vi "Create Electrode Array_2.vi"(7 "Current Channel":string, 8 "Insert\nBreak":bool=TRUE, 9 "Inverse\nPolarity":bool=TRUE, 10 "Electrode number, N":u16=100, 11 "Array Mode":u16(ring) items=["None", "Gradient + Dipole dipole", "Gradient", "Dipole Dipole", "Schlumberger"]) -> (3 "Current Mode":u8[][](array[numeric]))   [LabVIEW 2023]
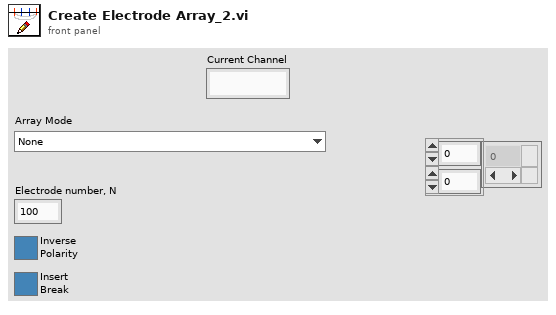
[diagram p1: front panel]
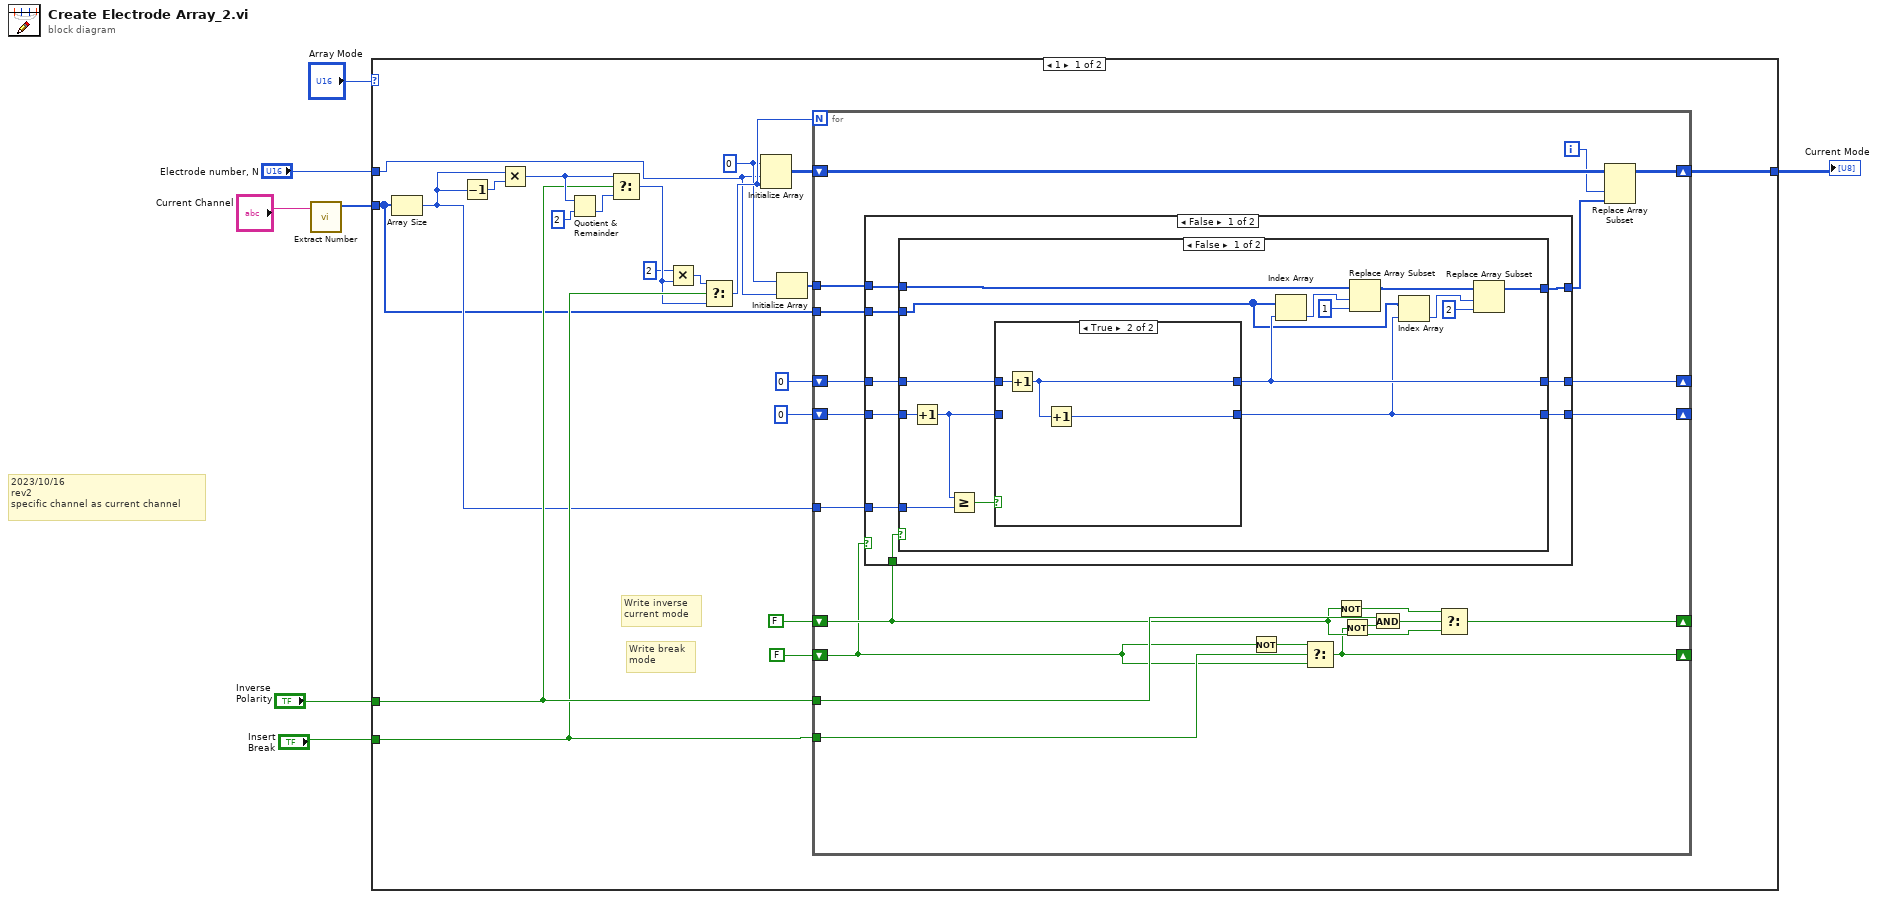
[diagram p0: block diagram]
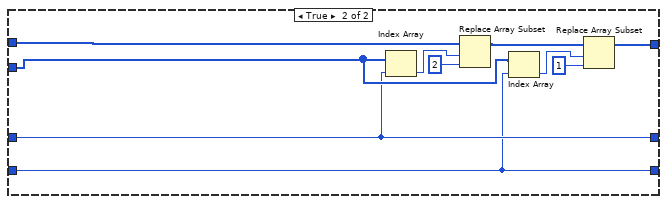
[diagram p3: hidden frame]
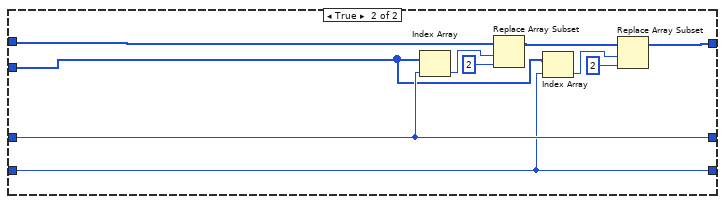
[diagram p4: hidden frame]
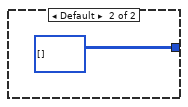
[diagram p5: hidden frame]
diagram:
  # "2023/10/16\nrev2 \nspecific channel as current channel"
  n1 = call "Extract Number.vi"("input string"="Current Channel") -> ("Array"=w1:i32[])  [unwired: 10 in]
  n2 = case shown="1" "Array Mode" {
    tunnel: "Electrode number, N" -> [w10 _]
    tunnel: "Inverse\nPolarity" -> [w18 _]
    tunnel: "Insert\nBreak" -> [w17 _]
    tunnel: [w14 u8[][] []] -> w3
    tunnel: w1 -> [w8 _]
    frame 1 {
      w15 = u8 0 ("stateArray")
      # "Write break\nmode"
      # "Write inverse\ncurrent mode"
      n3 = Array Size(array=w8) -> (size(s)=w9:i32)
      n4 = Decrement(x=w9) -> (x-1=w28:i32)
      n5 = Multiply(x=w9, y=w28) -> (x*y=w27:i32)
      n6 = Quotient & Remainder(x=w27, y=u16 2) -> (floor(x/y)=w25:i32)  [unwired: 1 out]
      n7 = Select(t=w27, s=w18, f=w25) -> (s? t:f=w12:i32)
      n8 = Multiply(x=u16 2, y=w12) -> (x*y=w13:i32)
      n9 = Select(t=w13, s=w17, f=w12) -> (s? t:f=w23:i32)
      n10 = Initialize Array(w15, w10, w23) -> (w24:u8[][])
      n11 = Initialize Array(w15, w10) -> (w16:u8[])
      n12 = for {
        N: w23 -> [_]
        shift-right: [w35] -> w14
        shift-left: w24 -> [w49]
        shift-right: [w38] -> _
        shift-left: 0 ("index (row)") -> [w41]
        shift-right: [w37] -> _
        shift-left: 0 ("index (row)") -> [w40]
        shift-right: [w45] -> _
        shift-left: FALSE ("Insert\nBreak") -> [w42]
        shift-right: [w32] -> _
        shift-left: FALSE ("Insert\nBreak") -> [w33]
        tunnel: w18 -> [w48]
        tunnel: w17 -> [w47]
        tunnel: w16 -> [w43]
        tunnel: w9 -> [w39]
        tunnel: w8 -> [w30]
        i -> [w44]
        n13 = case shown="False" w33 {
          tunnel: w43 -> [w57 w98]
          tunnel: [w54 w97] -> w36
          tunnel: w42 -> [w58 _]
          tunnel: w41 -> [w56 w96]
          tunnel: w40 -> [w55 w95]
          tunnel: w39 -> [w53 _]
          tunnel: [w52 w96] -> w38
          tunnel: [w51 w95] -> w37
          tunnel: w30 -> [w50 w94]
          frame False {
            n14 = case shown="False" w58 {
              tunnel: w57 -> [w73 w88]
              tunnel: w56 -> [w65 w80]
              tunnel: w55 -> [w68 w79]
              tunnel: [w69 w84] -> w54
              tunnel: w53 -> [w67 _]
              tunnel: [w63 w80] -> w52
              tunnel: [w60 w79] -> w51
              tunnel: w50 -> [w59 w81]
              frame False {
                n15 = Increment(x=w68) -> (x+1=w64:i32)
                n16 = Greater Or Equal?(x=w64, y=w67) -> (x >= y?=w66:bool)
                n17 = case shown="True" w66 {
                  tunnel: w65 -> [w74 w78]
                  tunnel: [w74 w77] -> w63
                  tunnel: [w75 w76] -> w60
                  tunnel: w64 -> [w75 _]
                  frame False {
                  }
                  frame True {
                    n18 = Increment(x=w78) -> (x+1=w77:i32)
                    n19 = Increment(x=w77) -> (x+1=w76:i32)
                  }
                }
                n20 = Index Array(array=w59, index=w63) -> (element=w62:i32)
                n21 = Replace Array Subset(array=w73, new element=u8 1 ("new element/subarray"), index=w62) -> (w70:u8[])
                n22 = Index Array(array=w59, index=w60) -> (element=w61:i32)
                n23 = Replace Array Subset(array=w70, new element=u8 2 ("new element/subarray"), index=w61) -> (w69:u8[])
              }
              frame True {
                n24 = Index Array(array=w81, index=w80) -> (element=w83:i32)
                n25 = Replace Array Subset(array=w88, new element=u8 2 ("new element/subarray"), index=w83) -> (w85:u8[])
                n26 = Index Array(array=w81, index=w79) -> (element=w82:i32)
                n27 = Replace Array Subset(array=w85, new element=u8 1 ("new element/subarray"), index=w82) -> (w84:u8[])
              }
            }
          }
          frame True {
            n28 = Index Array(array=w94, index=w96) -> (element=w90:i32)
            n29 = Replace Array Subset(array=w98, new element=u8 2 ("new element/subarray"), index=w90) -> (w91:u8[])
            n30 = Index Array(array=w94, index=w95) -> (element=w89:i32)
            n31 = Replace Array Subset(array=w91, new element=u8 2 ("new element/subarray"), index=w89) -> (w97:u8[])
          }
        }
        n32 = Not(x=w33) -> (.not. x?=w29:bool)
        n33 = Select(t=w29, s=w47, f=w33) -> (s? t:f=w32:bool)
        n34 = Not(x=w42) -> (.not. x?=w46:bool)
        n35 = Not(x=w32) -> (.not. x?=w31:bool)
        n36 = And(x=w48, y=w31) -> (x .and. y?=w34:bool)
        n37 = Select(t=w46, s=w34, f=w42) -> (s? t:f=w45:bool)
        n38 = Replace Array Subset(array=w49, new element=w36, index (col)=w44) -> (w35:u8[][])  [unwired: 1 in]
      }
    }
    frame Default {
    }
  }
  "Current Mode" <- w3
